vi "方程.vi"() -> ()   [LabVIEW 2018]
panel:
  out "结果":dbl
  in  "C":dbl
  in  "B":dbl
  in  "X":dbl
  in  "A":dbl
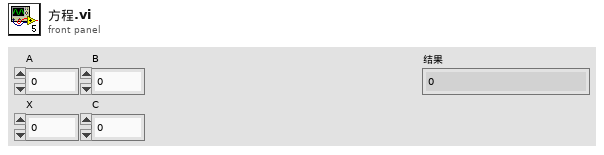
[diagram p1: front panel]
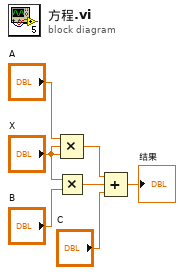
[diagram p0: block diagram]
diagram:
  n1 = Multiply(x="X", y="B") -> (x*y=w2:dbl)
  n2 = Compound Arithmetic op=MULTIPLY("A", "X", "X") -> (w3:dbl)
  n3 = Compound Arithmetic op=ADD(w3, w2, "C") -> (→"结果":dbl)
